vi "query range and autorange.vi"(8 "error in (no error)":errorcluster, 11 "VISA session":refnum<visa-resource-name>) -> (0 "error out":errorcluster, 1 "Auto Range (F: Off)":bool, 2 "Range (0: 1 - Lowest)":u16(ring) items=["1 - Lowest", "2", "3", "4", "5 - Highest"], 3 "dup VISA session":refnum<visa-resource-name>)   [LabVIEW 2017]
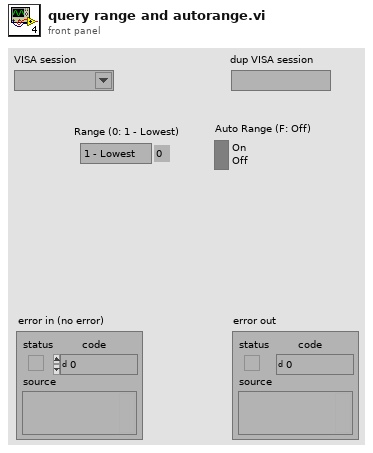
[diagram p1: front panel]
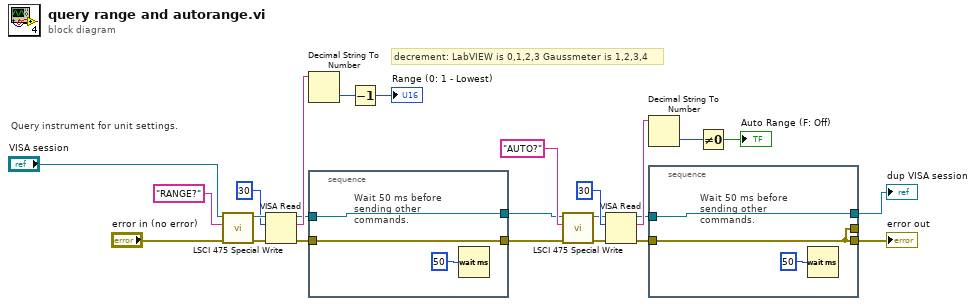
[diagram p0: block diagram]
diagram:
  # "decrement: LabVIEW is 0,1,2,3 Gaussmeter is 1,2,3,4"
  # "Query instrument for unit settings."
  n1 = call "LSCI 475 Special Write.vi"("error in (no error)"="error in (no error)", "Write Buffer (\"\")"="RANGE?", "VISA session"="VISA session") -> ("error out"=w21:errorcluster, "dup VISA session"=w22:refnum<visa-resource-name>)  [unwired: 6 in, 1 out]
  n2 = VISA Read(VISA resource name=w22, byte count=u32 30, error in (no error)=w21) -> (VISA resource name out=w9:refnum<visa-resource-name>, read buffer=w17:string, error out=w18:errorcluster)  [unwired: 1 out]
  n3 = Decimal String To Number(string=w17) -> (number=w16:i32)  [unwired: 2 in, 1 out]
  n4 = stacked-sequence {
    tunnel: w18 -> [w26]
    tunnel: [w26] -> w12
    tunnel: [w25] -> w10
    tunnel: w9 -> [w25]
    frame #0 {
      # "Wait 50 ms before\nsending other\ncommands."
      n5 = Wait (ms)(milliseconds to wait=u32 50) -> ()  [unwired: 1 out]
    }
  }
  n6 = Decrement(x=w16) -> (x-1=→"Range (0: 1 - Lowest)":i32)
  n7 = call "LSCI 475 Special Write.vi"("error in (no error)"=w12, "Write Buffer (\"\")"="AUTO?", "VISA session"=w10) -> ("error out"=w11:errorcluster, "dup VISA session"=w8:refnum<visa-resource-name>)  [unwired: 6 in, 1 out]
  n8 = VISA Read(VISA resource name=w8, byte count=u32 30, error in (no error)=w11) -> (VISA resource name out=w4:refnum<visa-resource-name>, read buffer=w7:string, error out=w3:errorcluster)  [unwired: 1 out]
  n9 = Decimal String To Number(string=w7) -> (number=w6:i32)  [unwired: 2 in, 1 out]
  n10 = stacked-sequence {
    tunnel: [w28] -> _
    tunnel: [w28] -> w1
    tunnel: [w29] -> w2
    tunnel: w4 -> [w29]
    tunnel: w3 -> [w28]
    frame #0 {
      # "Wait 50 ms before\nsending other\ncommands."
      n11 = Wait (ms)(milliseconds to wait=u32 50) -> ()  [unwired: 1 out]
    }
  }
  "dup VISA session" <- w2
  "error out" <- w1
  n12 = Not Equal To 0?(x=w6) -> (x != 0?=→"Auto Range (F: Off)":bool)
